vi "LEDBegin.vi"(8 "error in (no error)":errorcluster) -> (0 "error out":errorcluster)   [LabVIEW 2023]
uses:
  <vilib>/Rock Robotics/SystemInterfaces/DIO/FPGA_DIOChannel.ctl
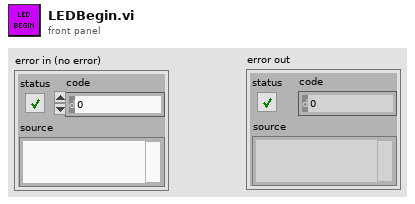
[diagram p1: front panel]
types:
  T1 = typedef "FPGA_DIOChannel.ctl" = enum8{"DIO 0", "DIO 1", "DIO 2", "DIO 3", "DIO 4", "DIO 5", "DIO 6", "DIO 7", "DIO 8", "DIO 9", "DIO MXP 0", "DIO MXP 1", "DIO MXP 2", "DIO MXP 3", "DIO MXP 4", "DIO MXP 5", "DIO MXP 6", "DIO MXP 7", "DIO MXP 8", "DIO MXP 9", "DIO MXP 10", "DIO MXP 11", "DIO MXP 12", "DIO MXP 13", "DIO MXP 14", "DIO MXP 15", "SPI Port CS1", "SPI Port CS2", "SPI Port CS3", "SPI Port MISO", "SPI Port MOSI", "Invalid"}
  T2 = typedef "WPI_DigitalOutputDevRef.ctl" = cluster{"DIO Channel":T1, "DevStatus":errorcluster}
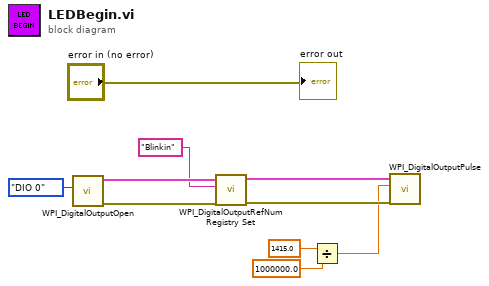
[diagram p0: block diagram]
diagram:
  n1 = call <vilib>:"WPI_DigitalOutputOpen.vi"("DIO Channel"=FPGA_DIOChannel."DIO 0") -> ("error out"=w6:errorcluster, "DigitalOutputDevRef"=w8:T2)  [unwired: 9 in]
  n2 = call <vilib>:"WPI_DigitalOutputRefNum Registry Set.vi"("error in (no error)"=w6, "refnum name"="Blinkin", "DigitalOutputDevRef"=w8) -> ("error out"=w4:errorcluster, "DigitalOutputDevRef"=w5:T2)  [unwired: 7 in]
  n3 = Divide(x=1415.0, y=1000000.0) -> (x/y=w2:dbl)
  n4 = call <vilib>:"WPI_DigitalOutputPulse.vi"("error in (no error)"=w4, "length (Sec)"=w2, "DigitalOutputDevRef"=w5) -> ()  [unwired: 7 in, 2 out]
  "error out" <- "error in (no error)"
